vi "EQ.vi"(8 "error in (no error)":errorcluster, 10 "Audio Block In":dbl[][](array[numeric]), 11 "Channel in":refnum<class "Channel.lvclass">) -> (0 "error out":errorcluster, 2 "Audio Block Out":dbl[][](array[numeric]))   [LabVIEW 2018, in "Channel.lvclass"]
doc: "Perform 3-band (low, mid, high) equalization of the audio data using Butterworth filters."
uses:
  Channel.lvclass
  Channel.lvclass/Channel.ctl
  <vilib>/Analysis/3filter.llb/Filter Passband Type.ctl
  Libraries/Globals/Constants.vi
  <vilib>/Analysis/3filter.llb/Butterworth Filter (DBL).vi
  <vilib>/Analysis/NI_AALBase.lvlib
  Libraries/Globals/Globals.lvlib
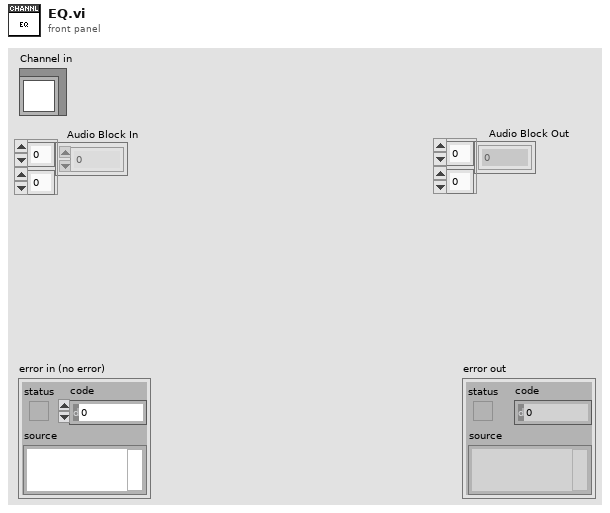
[diagram p1: front panel]
types:
  T1 = typedef "NI_AALBase.lvlib/Filter Passband Type.ctl" = enum32{"Lowpass", "Highpass", "Bandpass", "Bandstop"}
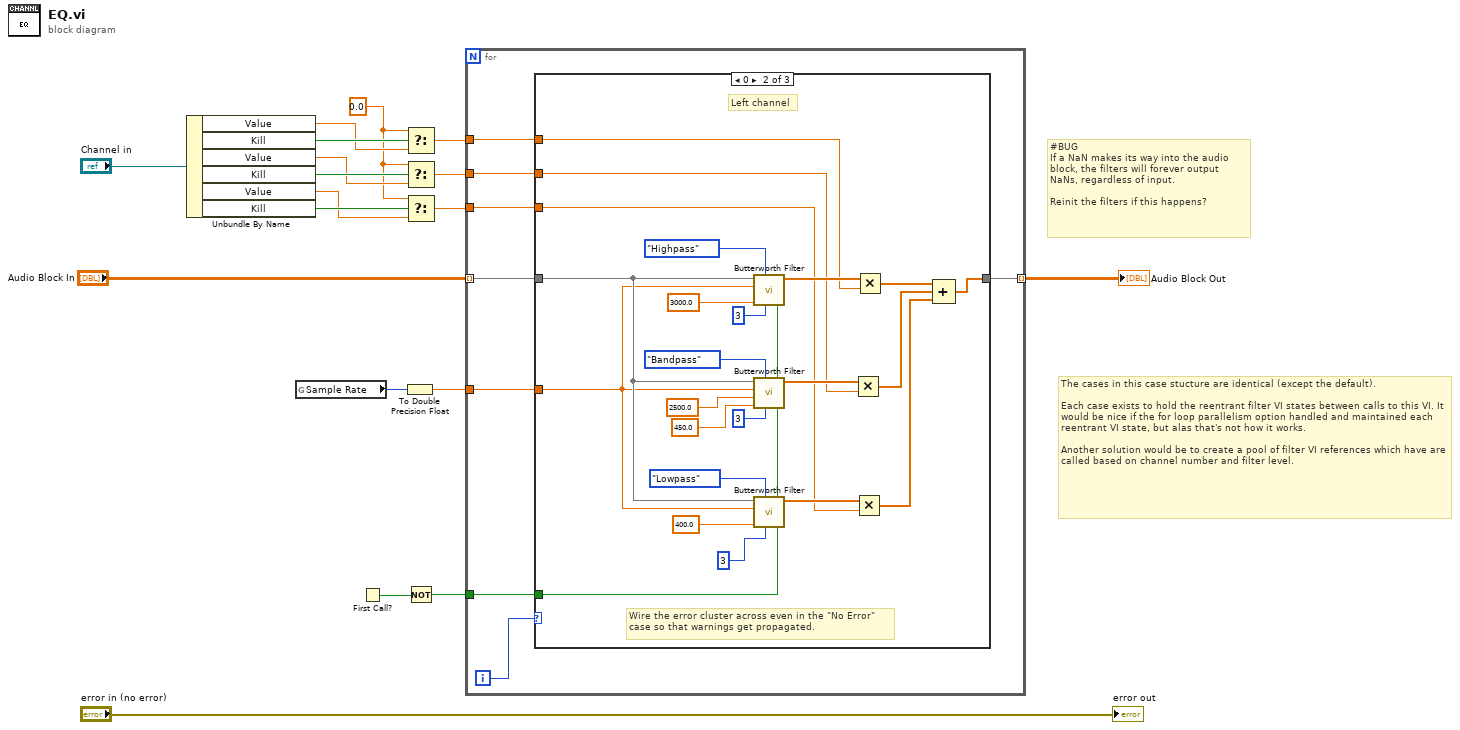
[diagram p0: block diagram]
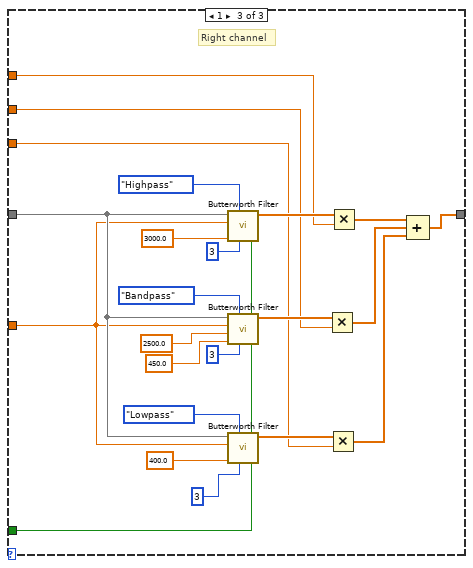
[diagram p3: hidden frame]
diagram:
  w10 = 0.0 ("t")
  # "#BUG\nIf a NaN makes its way into the audio block, the filters will forever output NaNs, regardless of input.\n\nReinit the filters if this happens?"
  # "Wire the error cluster across even in the \"No Error\"\ncase so that warnings get propagated."
  # "The cases in this case stucture are identical (except the default).\n\nEach case exists to hold the reentrant filter VI states between calls to this VI. It would be nice if the for loop parallelism option handled and maintained each reentrant VI state, but alas that's not how it works.\n\nAnother solution would be to create a pool of filter VI references which have are called based on channel number and filter level."
  n1 = Unbundle By Name("Channel in") -> ("Value"=w13:dbl, "Kill"=w14:bool, "Value"=w11:dbl, "Kill"=w12:bool, "Value"=w8:dbl, "Kill"=w9:bool)
  n2 = global read "Constants.vi" "Sample Rate"() -> (w2:i32)
  n3 = First Call?() -> (First Call?: T/F=w4:bool)
  n4 = To Double Precision Float(number=w2) -> (double precision float=w1:dbl)
  n5 = Select(t=w10, s=w14, f=w13) -> (s? t:f=w7:dbl)
  n6 = Select(t=w10, s=w12, f=w11) -> (s? t:f=w6:dbl)
  n7 = Select(t=w10, s=w9, f=w8) -> (s? t:f=w5:dbl)
  n8 = Not(x=w4) -> (.not. x?=w3:bool)
  n9 = for {
    tunnel: "Audio Block In" -> [w26] mode=indexing
    tunnel: w5 -> [w25]
    tunnel: w6 -> [w24]
    tunnel: w7 -> [w23]
    tunnel: [w22] -> w15 mode=indexing
    tunnel: w3 -> [w21]
    tunnel: w1 -> [w19]
    i -> [w20]
    n10 = case shown="0" w20 {
      tunnel: w26 -> [w27 w37 w60]
      tunnel: w25 -> [_ w36 w59]
      tunnel: w24 -> [_ w35 w58]
      tunnel: w23 -> [_ w34 w57]
      tunnel: [w27 w33 w56] -> w22
      tunnel: w21 -> [_ w32 w55]
      tunnel: w19 -> [_ w28 w51]
      frame Default {
        # "Not expecting more than two channels, so pass them through unfiltered"
      }
      frame 0 {
        # "Left channel"
        n11 = call-poly <vilib>:"Butterworth Filter.vi"("init/cont (init:F)"=w32, "order"=3, "filter type"=Filter_Passband_Type."Highpass", "low cutoff freq: fl"=3000.0 ("high cutoff freq: fh"), "sampling freq: fs"=w28, "X"=w37) -> ("Filtered X"=w45:dbl[])  [unwired: 2 in, 1 out]
        n12 = call-poly <vilib>:"Butterworth Filter.vi"("init/cont (init:F)"=w32, "order"=3, "filter type"=Filter_Passband_Type."Bandpass", "low cutoff freq: fl"=450.0, "high cutoff freq: fh"=2500.0, "sampling freq: fs"=w28, "X"=w37) -> ("Filtered X"=w43:dbl[])  [unwired: 1 in, 1 out]
        n13 = call-poly <vilib>:"Butterworth Filter.vi"("init/cont (init:F)"=w32, "order"=3, "filter type"=Filter_Passband_Type."Lowpass", "low cutoff freq: fl"=400.0, "sampling freq: fs"=w28, "X"=w37) -> ("Filtered X"=w41:dbl[])  [unwired: 2 in, 1 out]
        n14 = Multiply(x=w43, y=w35) -> (x*y=w42:dbl[])
        n15 = Multiply(x=w41, y=w36) -> (x*y=w40:dbl[])
        n16 = Multiply(x=w45, y=w34) -> (x*y=w44:dbl[])
        n17 = Compound Arithmetic op=ADD(w44, w42, w40) -> (w33:dbl[])
      }
      frame 1 {
        # "Right channel"
        n18 = call-poly <vilib>:"Butterworth Filter.vi"("init/cont (init:F)"=w55, "order"=3, "filter type"=Filter_Passband_Type."Highpass", "low cutoff freq: fl"=3000.0 ("high cutoff freq: fh"), "sampling freq: fs"=w51, "X"=w60) -> ("Filtered X"=w68:dbl[])  [unwired: 2 in, 1 out]
        n19 = call-poly <vilib>:"Butterworth Filter.vi"("init/cont (init:F)"=w55, "order"=3, "filter type"=Filter_Passband_Type."Bandpass", "low cutoff freq: fl"=450.0, "high cutoff freq: fh"=2500.0, "sampling freq: fs"=w51, "X"=w60) -> ("Filtered X"=w66:dbl[])  [unwired: 1 in, 1 out]
        n20 = call-poly <vilib>:"Butterworth Filter.vi"("init/cont (init:F)"=w55, "order"=3, "filter type"=Filter_Passband_Type."Lowpass", "low cutoff freq: fl"=400.0, "sampling freq: fs"=w51, "X"=w60) -> ("Filtered X"=w64:dbl[])  [unwired: 2 in, 1 out]
        n21 = Multiply(x=w66, y=w58) -> (x*y=w65:dbl[])
        n22 = Multiply(x=w64, y=w59) -> (x*y=w63:dbl[])
        n23 = Multiply(x=w68, y=w57) -> (x*y=w67:dbl[])
        n24 = Compound Arithmetic op=ADD(w67, w65, w63) -> (w56:dbl[])
      }
    }
  }
  "Audio Block Out" <- w15
  "error out" <- "error in (no error)"
